vi "Initialize Unit Ring Control.vi"(9 "Value":u16, 10 "Quantity":T1=enum."Acceleration", 11 "Ctrl Ref":refnum<vi>) -> ()   [LabVIEW 2011]
uses:
  Quantity enum.ctl
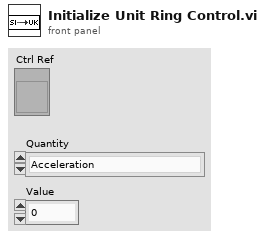
[diagram p1: front panel]
types:
  T1 = typedef "Quantity enum.ctl" = enum16{"NA", "Acceleration", "Angle", "Current", "Force", "Distance", "Pressure", "Resistance", "Rotational Speed", "Speed", "Temperature", "Tension", "Torque", "Voltage", "Weight"}
  T2 = cluster{"Available Units":cluster{"Unit":string, "Gain":dbl, "Offset":dbl}[]}[]
  T3 = cluster{"Available Units":cluster{"Unit":string, "Gain":dbl, "Offset":dbl}[]}
  T4 = cluster{"Unit":string, "Gain":dbl, "Offset":dbl}[]
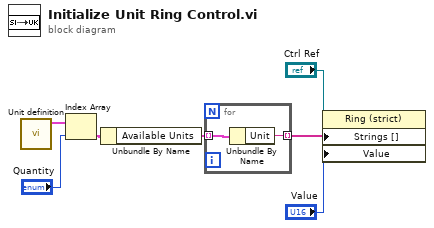
[diagram p0: block diagram]
diagram:
  n1 = call "Unit definition.vi"() -> ("Array"=w7:T2)  [unwired: 11 in]
  n2 = Index Array(array=w7, index="Quantity") -> (element=w6:T3)
  n3 = Unbundle By Name(w6) -> ("Available Units"=w5:T4)
  n4 = for {
    tunnel: w5 -> [w9] mode=indexing
    tunnel: [w8] -> w3 mode=indexing
    n5 = Unbundle By Name(w9) -> ("Unit"=w8:string)
  }
  n6 = property on="Property Node" class="Ring (strict)"(reference="Ctrl Ref", "Strings []"=w3, "Value"="Value") -> ()  [unwired: 1 in, 2 out]
